vi "Untitled 1.vi"() -> ()   [LabVIEW 2018]
panel:
  in  "milliseconds to wait":u32
  out "Boolean":bool
  out "Button Input 2":bool
  in  "Button Input":bool
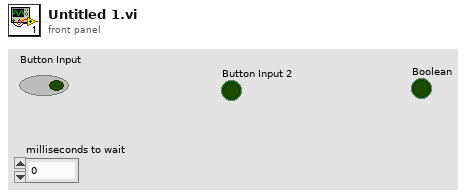
[diagram p1: front panel]
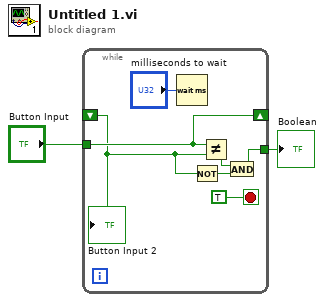
[diagram p0: block diagram]
diagram:
  n1 = while {
    shift-right: [w9] -> _
    shift-left: _ -> [w5]
    tunnel: "Button Input" -> [w9]
    tunnel: [w3] -> w1
    stop <- TRUE stop-if-true
    n2 = Wait (ms)(milliseconds to wait="milliseconds to wait") -> ()  [unwired: 1 out]
    n3 = Not(x=w5) -> (.not. x?=w4:bool)
    n4 = Not Equal?(x=w9, y=w5) -> (x != y?=w6:bool)
    n5 = And(x=w6, y=w4) -> (x .and. y?=w3:bool)
    "Button Input 2" <- w5
  }
  "Boolean" <- w1
